vi "Actividad_Labview.vi"() -> ()   [LabVIEW 2020]
uses:
  <vilib>/Motion/Express/_s/nimc.fb.straightLineMove.startStraightLineMove.axis.modeRelative.0.vi
  <vilib>/Motion/BlockNode/FB.NIMotion.xnode
panel:
  in  "position 4":dbl
  out "done 4":bool
  in  "execute 4":bool
  in  "position 3":dbl
  out "done 3":bool
  in  "execute 3":bool
  in  "position 2":dbl
  out "done 2":bool
  in  "execute 2":bool
  in  "stop":bool
  in  "position":dbl
  out "done":bool
  in  "execute":bool
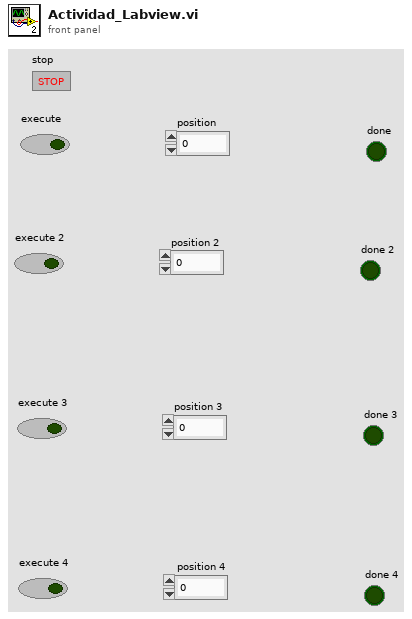
[diagram p1: front panel]
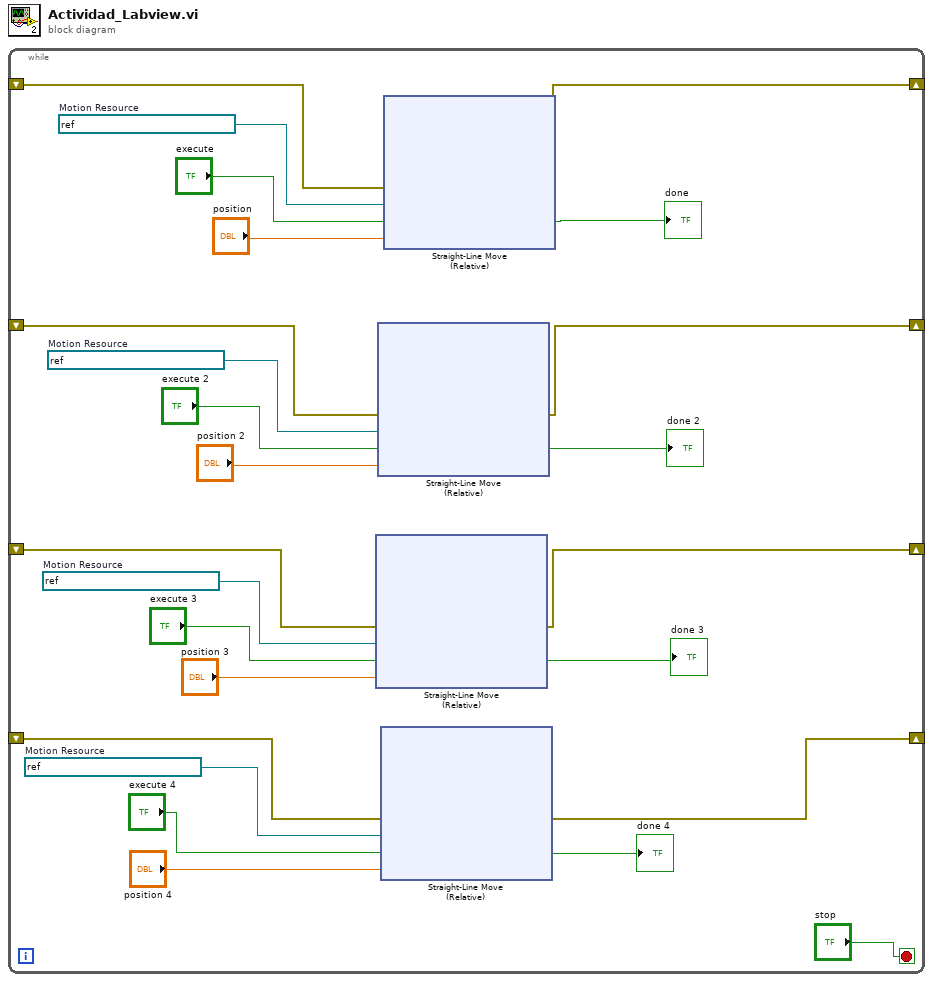
[diagram p0: block diagram]
diagram:
  n1 = while {
    shift-right: [w11] -> _
    shift-left: _ -> [w12]
    shift-right: [w7] -> _
    shift-left: _ -> [w8]
    shift-right: [w4] -> _
    shift-left: _ -> [w5]
    shift-right: [w1] -> _
    shift-left: _ -> [w2]
    stop <- "stop" stop-if-true
    w13 = refnum<k21> "nism://My Computer/Axis 4"  # Motion Resource
    w9 = refnum<k21> "nism://My Computer/Axis 3"  # Motion Resource
    w6 = refnum<k21> "nism://My Computer/Axis 2"  # Motion Resource
    w3 = refnum<k21> "nism://My Computer/Axis 1"  # Motion Resource
    n2 = xnode "Straight-Line Move\n(Relative)"("error in"=w8, "resource"=w9, "execute"="execute 3", "position"="position 3") -> ("error out"=w7:errorcluster, "done"=→"done 3":bool)  [unwired: 1 out]
    n3 = xnode "Straight-Line Move\n(Relative)"("error in"=w5, "resource"=w6, "execute"="execute 2", "position"="position 2") -> ("error out"=w4:errorcluster, "done"=→"done 2":bool)  [unwired: 1 out]
    n4 = xnode "Straight-Line Move\n(Relative)"("error in"=w12, "resource"=w13, "execute"="execute 4", "position"="position 4") -> ("error out"=w11:errorcluster, "done"=→"done 4":bool)  [unwired: 1 out]
    n5 = xnode "Straight-Line Move\n(Relative)"("error in"=w2, "resource"=w3, "execute"="execute", "position"="position") -> ("error out"=w1:errorcluster, "done"=→"done":bool)  [unwired: 1 out]
  }
